vi "Valve_EPICS_Dev4_APX.vi"() -> ()   [LabVIEW 2015]
uses:
  <userlib>/caLab/Private/Get_PV-1D.vi
  <userlib>/caLab/Private/Put_DBL-1D_PV-1D.vi
panel:
  out "Status":bool
  out "Numeric":i32
  out "APX:V7_CLOSE_REQ":bool
  out "APX:V6_CLOSE_REQ":bool
  out "APX:V5_CLOSE_REQ":bool
  out "APX:V4_CLOsE_REQ":bool
  out "AXP:V3_CLOSE_REQ":bool
  out "APX:V2_CLOSE_REQ":bool
  out "APX:V1_CLOSE_REQ":bool
  out "APX:V0_CLOSE_REQ":bool
  out "APX:V7_OPEN_REQ":bool
  out "APX:V6_OPEN_REQ":bool
  out "APX:V5_OPEN_REQ":bool
  out "APX:V4_OPEN_REQ":bool
  out "AXP:V3_OPEN_REQ":bool
  out "APX:V2_OPEN_REQ":bool
  out "APX:V1_OPEN_REQ":bool
  out "APX:V0_OPEN_REQ":bool
  out "APX:V7_OPEN_ENB":bool
  out "APX:V6_OPEN_ENB":bool
  out "APX:V5_OPEN_ENB":bool
  out "APX:V4_OPEN_ENB":bool
  out "APX:V3_OPEN_ENB":bool
  out "APX:V2_OPEN_ENB":bool
  out "APX:V1_OPEN_ENB":bool
  out "APX:V0_OPEN_ENB":bool
  out "Boolean array":bool[](array[boolean])
  out "APX:V7_OPEN_ACT":bool
  out "APX:V6_OPEN_ACT":bool
  out "APX:V5_OPEN_ACT":bool
  out "APX:V4_OPEN_ACT":bool
  out "APX:V3_OPEN_ACT":bool
  out "APX:V2_OPEN_ACT":bool
  out "APX:V1_OPEN_ACT":bool
  out "APX:V0_OPEN_ACT":bool
  out "initialized array":i16[](array[numeric])
  in  "stop":bool
  out "sum":i16
  out "0, 1":i16[](array[numeric])
  out "SCL_data":u32[](array[numeric]) caption="SCL"
  out "SOP_data":u32[](array[numeric]) caption="SOP"
  out "APX:V7_SCL":bool
  out "APX:V6_SCL":bool
  out "APX:V5_SCL":bool
  out "APX:V4_SCL":bool
  out "APX:V3_SCL":bool
  out "APX:V2_SCL":bool
  out "APX:V1_SCL":bool
  out "APX:V0_SCL":bool
  out "APX:V7_SOP":bool
  out "APX:V6_SOP":bool
  out "APX:V5_SOP":bool
  out "APX:V4_SOP":bool
  out "APX:V3_SOP":bool
  out "APX:V2_SOP":bool
  out "APX:V1_SOP":bool
  out "APX:V0_SOP":bool
  # "Valve control DEV4"
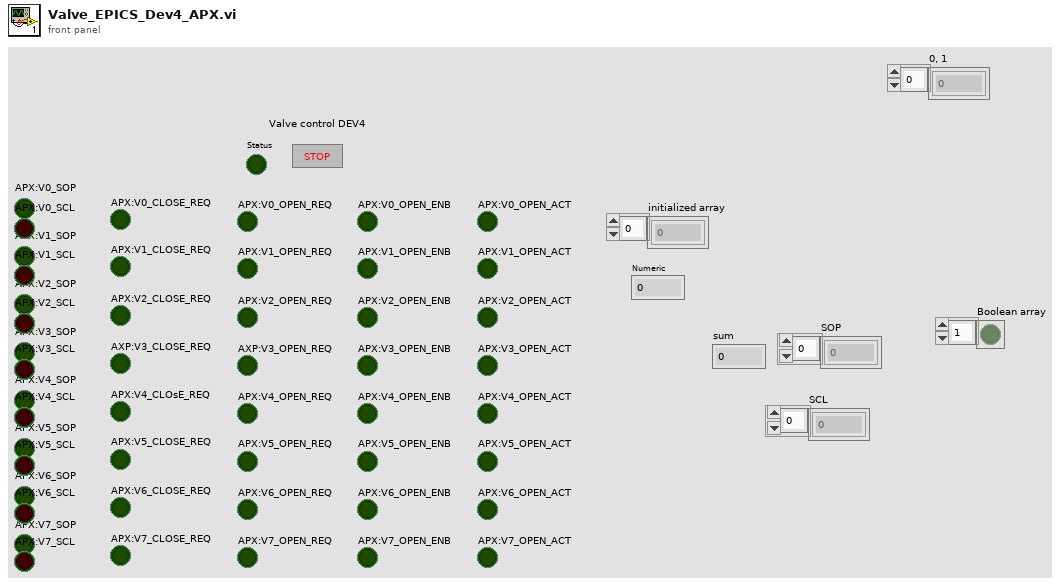
[diagram p1: front panel]
types:
  T1 = typedef "NI_Matrix.lvlib/RealMatrix.ctl" = dbl[][]
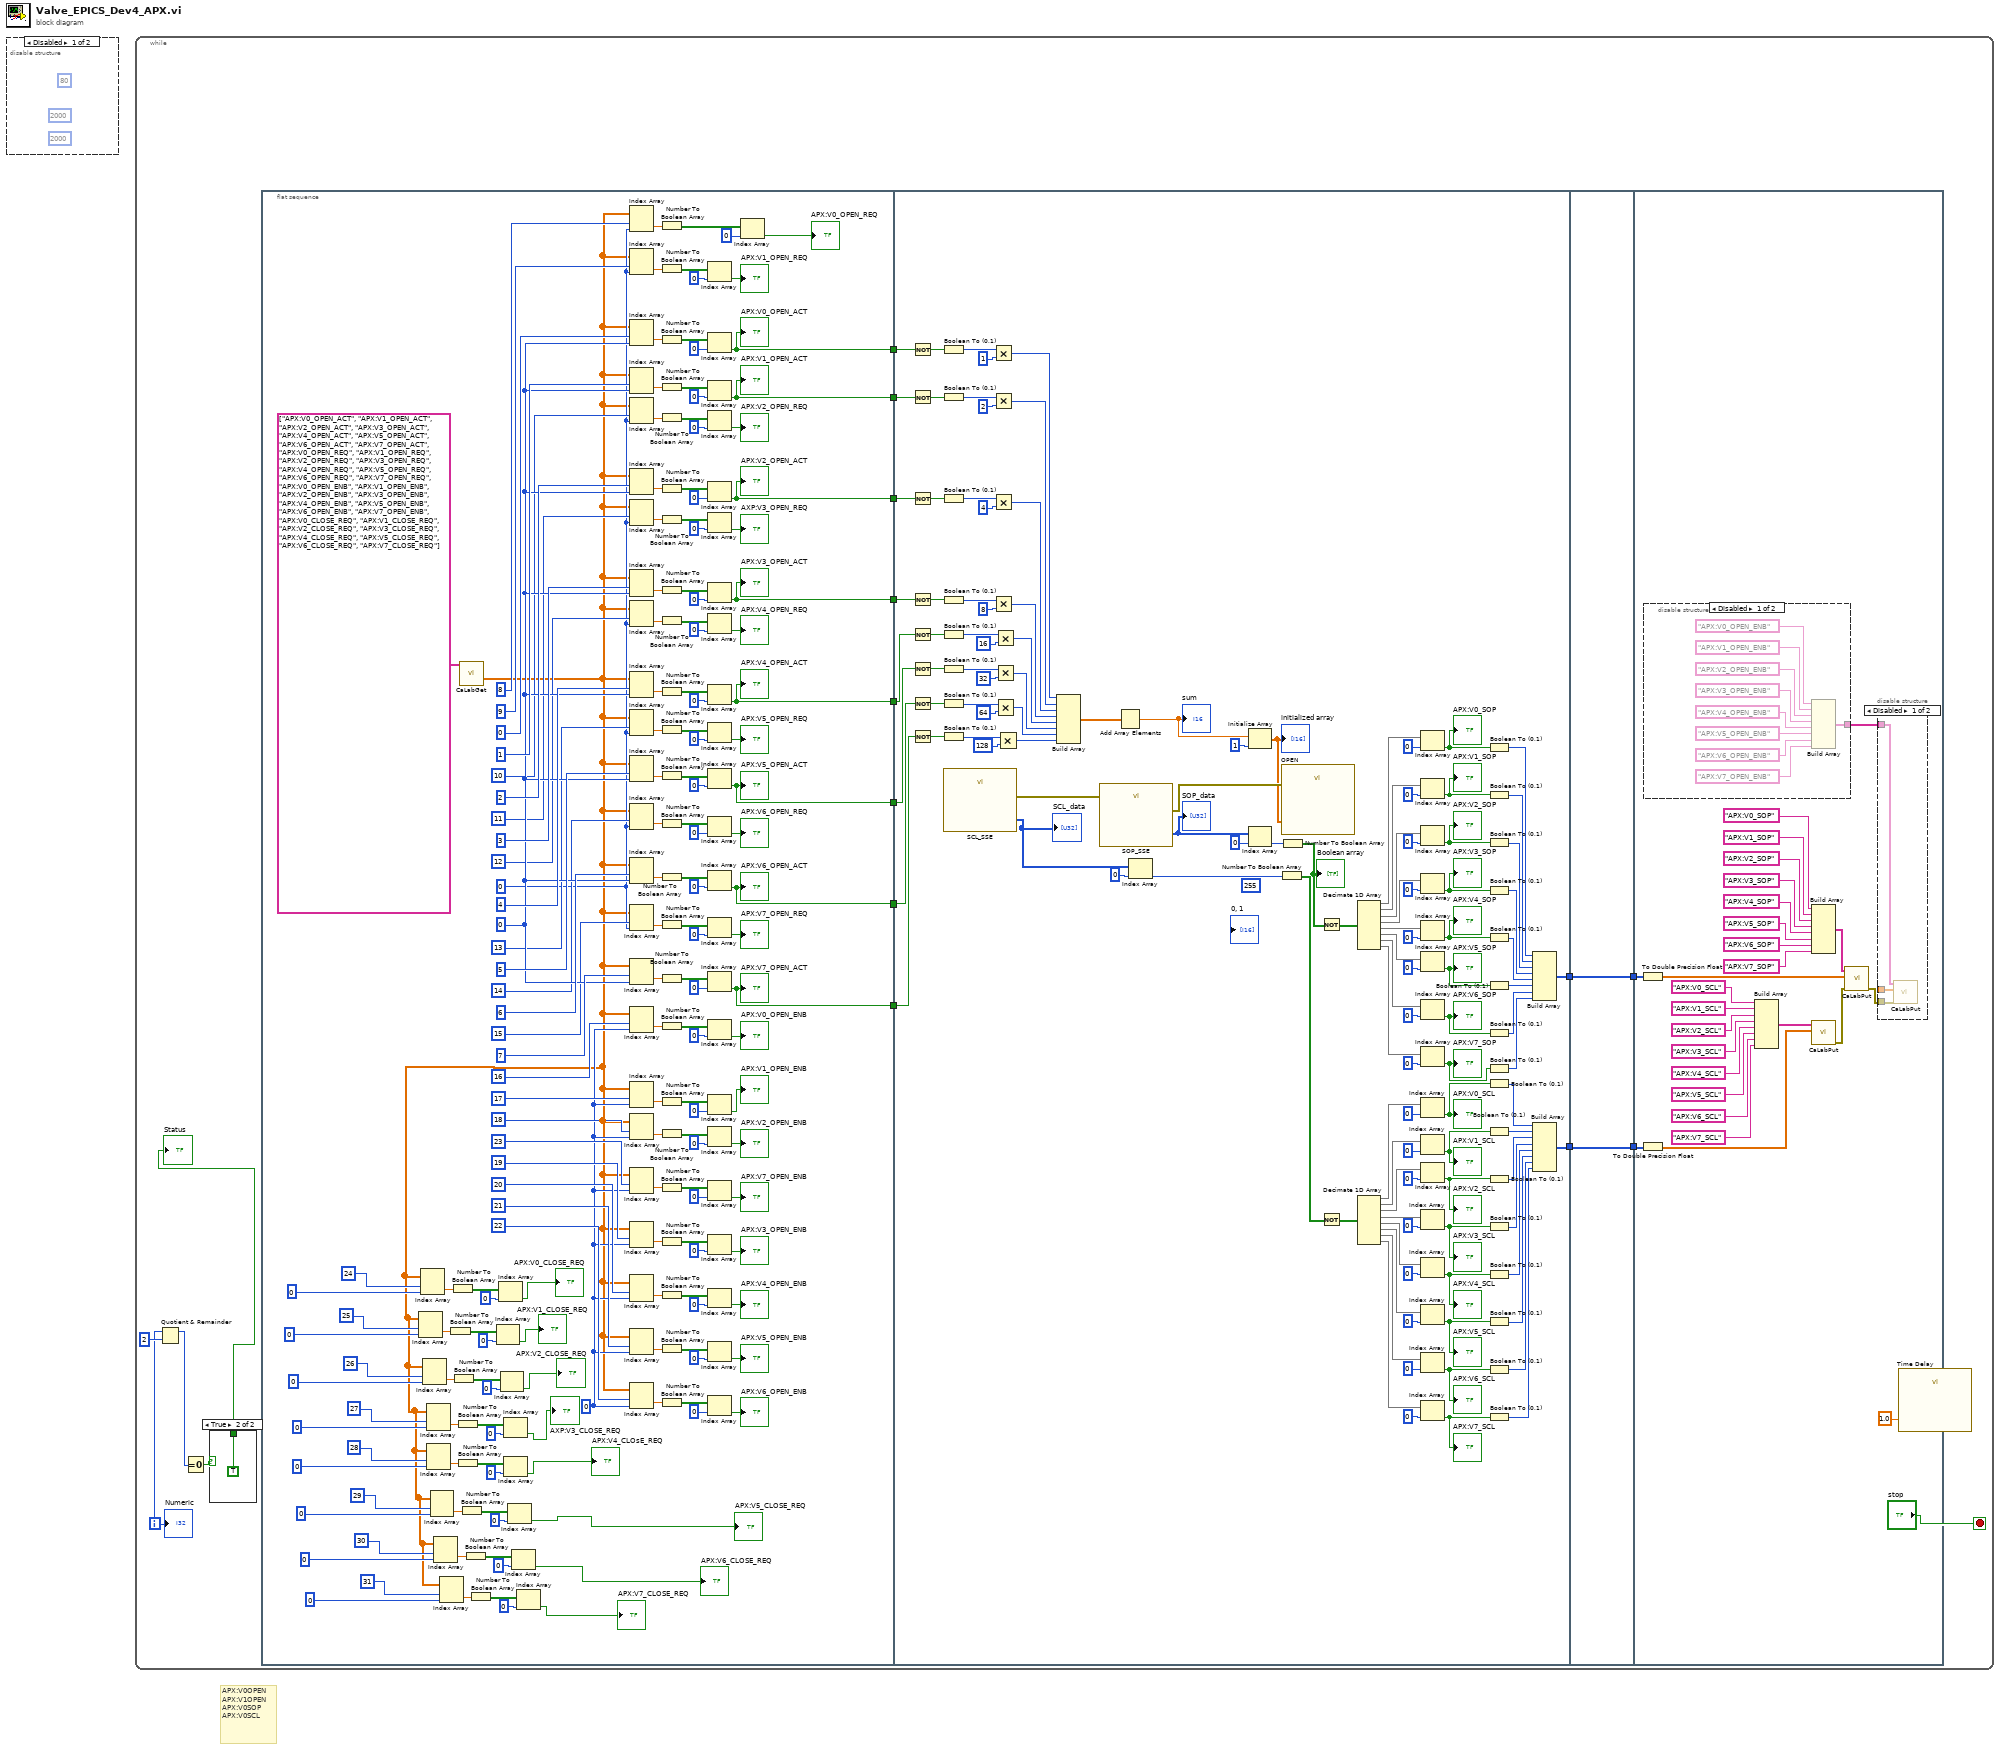
[diagram p0: block diagram]
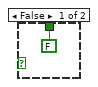
[diagram p3: hidden frame]
diagram:
  # "APX:V0OPEN\nAPX:V1OPEN\nAPX:V0SOP\nAPX:V0SCL"
  n1 = disable-structure shown="Disabled" {
    frame Disabled {
      w1 = 80 ("Priority")
      w2 = 2000 ("Timeout")
      w3 = i64 2000 ("Deadline")
    }
    frame Enabled {
    }
  }
  n2 = while {
    i -> [w5]
    stop <- "stop" stop-if-true
    n3 = Quotient & Remainder(x=w5, y=2) -> (x-y*floor(x/y)=w7:i32)  [unwired: 1 out]
    n4 = Equal To 0?(x=w7) -> (x = 0?=w8:bool)
    n5 = case shown="True" w8 {
      tunnel: [FALSE ("Status") TRUE ("Status")] -> w4
      frame False {
      }
      frame True {
      }
    }
    "Status" <- w4
    n6 = flat-sequence {
      tunnel: [w80] -> w22
      tunnel: [w79] -> w21
      tunnel: [w75] -> w20
      tunnel: [w82] -> w19
      tunnel: [w81] -> w18
      tunnel: [w78] -> w17
      tunnel: [w77] -> w16
      tunnel: [w76] -> w15
      tunnel: w22 -> [w256]
      tunnel: w21 -> [w257]
      tunnel: w20 -> [w258]
      tunnel: w19 -> [w263]
      tunnel: w18 -> [w255]
      tunnel: w17 -> [w259]
      tunnel: w16 -> [w260]
      tunnel: w15 -> [w261]
      tunnel: [w207] -> w14
      tunnel: [w296] -> w11
      tunnel: w14 -> [w321]
      tunnel: [w321] -> w13
      tunnel: w11 -> [w320]
      tunnel: [w320] -> w10
      tunnel: w13 -> [w328]
      tunnel: w10 -> [w326]
      frame #0 {
        w74 = 0 ("index")
        w155 = 0 ("index")
        w188 = 0 ("index")
        n7 = call-poly "CaLabGet.vi"("PV Names"=string[] ["APX:V0_OPEN_ACT", "APX:V1_OPEN_ACT", "APX:V2_OPEN_ACT", "APX:V3_OPEN_ACT", "APX:V4_OPEN_ACT", "APX:V5_OPEN_ACT", "APX:V6_OPEN_ACT", "APX:V7_OPEN_ACT", "APX:V0_OPEN_REQ", "APX:V1_OPEN_REQ", "APX:V2_OPEN_REQ", "APX:V3_OPEN_REQ", "APX:V4_OPEN_REQ", "APX:V5_OPEN_REQ", "APX:V6_OPEN_REQ", "APX:V7_OPEN_REQ", "APX:V0_OPEN_ENB", "APX:V1_OPEN_ENB", "APX:V2_OPEN_ENB", "APX:V3_OPEN_ENB", "APX:V4_OPEN_ENB", "APX:V5_OPEN_ENB", "APX:V6_OPEN_ENB", "APX:V7_OPEN_ENB", "APX:V0_CLOSE_REQ", "APX:V1_CLOSE_REQ", "APX:V2_CLOSE_REQ", "APX:V3_CLOSE_REQ", "APX:V4_CLOSE_REQ", "APX:V5_CLOSE_REQ", "APX:V6_CLOSE_REQ", "APX:V7_CLOSE_REQ"]) -> ("Value Array (number)"=w33:dbl[][])  [unwired: 8 in, 6 out]
        n8 = Index Array(array=w33, index (row)=25 ("index"), index (col)=0 ("index")) -> (element=w66:dbl)
        n9 = Index Array(array=w33, index (row)=24 ("index"), index (col)=0 ("index")) -> (element=w71:dbl)
        n10 = Index Array(array=w33, index (row)=26 ("index"), index (col)=0 ("index")) -> (element=w61:dbl)
        n11 = Index Array(array=w33, index (row)=27 ("index"), index (col)=0 ("index")) -> (element=w56:dbl)
        n12 = Index Array(array=w33, index (row)=28 ("index"), index (col)=0 ("index")) -> (element=w51:dbl)
        n13 = Index Array(array=w33, index (row)=29 ("index"), index (col)=0 ("index")) -> (element=w46:dbl)
        n14 = Index Array(array=w33, index (row)=30 ("index"), index (col)=0 ("index")) -> (element=w41:dbl)
        n15 = Index Array(array=w33, index (row)=31 ("index"), index (col)=0 ("index")) -> (element=w36:dbl)
        n16 = Number To Boolean Array(number=w66) -> (Boolean array=w68:bool[])
        n17 = Number To Boolean Array(number=w71) -> (Boolean array=w73:bool[])
        n18 = Number To Boolean Array(number=w61) -> (Boolean array=w63:bool[])
        n19 = Number To Boolean Array(number=w56) -> (Boolean array=w58:bool[])
        n20 = Number To Boolean Array(number=w51) -> (Boolean array=w53:bool[])
        n21 = Number To Boolean Array(number=w46) -> (Boolean array=w48:bool[])
        n22 = Number To Boolean Array(number=w41) -> (Boolean array=w43:bool[])
        n23 = Number To Boolean Array(number=w36) -> (Boolean array=w38:bool[])
        n24 = Index Array(array=w68, index=0) -> (element=→"APX:V1_CLOSE_REQ":bool)
        n25 = Index Array(array=w73, index=0) -> (element=→"APX:V0_CLOSE_REQ":bool)
        n26 = Index Array(array=w63, index=0) -> (element=→"APX:V2_CLOSE_REQ":bool)
        n27 = Index Array(array=w58, index=0) -> (element=→"AXP:V3_CLOSE_REQ":bool)
        n28 = Index Array(array=w53, index=0) -> (element=→"APX:V4_CLOsE_REQ":bool)
        n29 = Index Array(array=w48, index=0) -> (element=→"APX:V5_CLOSE_REQ":bool)
        n30 = Index Array(array=w43, index=0) -> (element=→"APX:V6_CLOSE_REQ":bool)
        n31 = Index Array(array=w38, index=0) -> (element=→"APX:V7_CLOSE_REQ":bool)
        n32 = Index Array(array=w33, index (row)=8 ("disabled index (row)"), index (col)=w155) -> (element=w135:dbl)
        n33 = Index Array(array=w33, index (row)=9, index (col)=w155) -> (element=w134:dbl)
        n34 = Index Array(array=w33, index (row)=0 ("disabled index (row)"), index (col)=w188) -> (element=w168:dbl)
        n35 = Index Array(array=w33, index (row)=1, index (col)=w188) -> (element=w167:dbl)
        n36 = Index Array(array=w33, index (row)=10, index (col)=w155) -> (element=w138:dbl)
        n37 = Index Array(array=w33, index (row)=2, index (col)=w188) -> (element=w171:dbl)
        n38 = Index Array(array=w33, index (row)=11 ("index"), index (col)=w155) -> (element=w137:dbl)
        n39 = Index Array(array=w33, index (row)=3 ("index"), index (col)=w188) -> (element=w170:dbl)
        n40 = Index Array(array=w33, index (row)=12, index (col)=w155) -> (element=w136:dbl)
        n41 = Index Array(array=w33, index (row)=4, index (col)=w188) -> (element=w169:dbl)
        n42 = Index Array(array=w33, index (row)=13, index (col)=w155) -> (element=w133:dbl)
        n43 = Index Array(array=w33, index (row)=5, index (col)=w188) -> (element=w166:dbl)
        n44 = Index Array(array=w33, index (row)=14, index (col)=w155) -> (element=w132:dbl)
        n45 = Index Array(array=w33, index (row)=6, index (col)=w188) -> (element=w165:dbl)
        n46 = Index Array(array=w33, index (row)=15, index (col)=w155) -> (element=w131:dbl)
        n47 = Index Array(array=w33, index (row)=7, index (col)=w188) -> (element=w164:dbl)
        n48 = Index Array(array=w33, index (row)=16 ("disabled index (row)"), index (col)=w74) -> (element=w103:dbl)
        n49 = Index Array(array=w33, index (row)=17, index (col)=w74) -> (element=w102:dbl)
        n50 = Index Array(array=w33, index (row)=18, index (col)=w74) -> (element=w106:dbl)
        n51 = Index Array(array=w33, index (row)=23, index (col)=w74) -> (element=w99:dbl)
        n52 = Index Array(array=w33, index (row)=19 ("index"), index (col)=w74) -> (element=w105:dbl)
        n53 = Index Array(array=w33, index (row)=20, index (col)=w74) -> (element=w104:dbl)
        n54 = Index Array(array=w33, index (row)=21, index (col)=w74) -> (element=w101:dbl)
        n55 = Index Array(array=w33, index (row)=22, index (col)=w74) -> (element=w100:dbl)
        n56 = Number To Boolean Array(number=w135) -> (Boolean array=w148:bool[])
        n57 = Number To Boolean Array(number=w134) -> (Boolean array=w146:bool[])
        n58 = Number To Boolean Array(number=w168) -> (Boolean array=w181:bool[])
        n59 = Number To Boolean Array(number=w167) -> (Boolean array=w179:bool[])
        n60 = Number To Boolean Array(number=w138) -> (Boolean array=w154:bool[])
        n61 = Number To Boolean Array(number=w171) -> (Boolean array=w187:bool[])
        n62 = Number To Boolean Array(number=w137) -> (Boolean array=w152:bool[])
        n63 = Number To Boolean Array(number=w170) -> (Boolean array=w185:bool[])
        n64 = Number To Boolean Array(number=w136) -> (Boolean array=w150:bool[])
        n65 = Number To Boolean Array(number=w169) -> (Boolean array=w183:bool[])
        n66 = Number To Boolean Array(number=w133) -> (Boolean array=w144:bool[])
        n67 = Number To Boolean Array(number=w166) -> (Boolean array=w177:bool[])
        n68 = Number To Boolean Array(number=w132) -> (Boolean array=w142:bool[])
        n69 = Number To Boolean Array(number=w165) -> (Boolean array=w175:bool[])
        n70 = Number To Boolean Array(number=w131) -> (Boolean array=w140:bool[])
        n71 = Number To Boolean Array(number=w164) -> (Boolean array=w173:bool[])
        n72 = Number To Boolean Array(number=w103) -> (Boolean array=w116:bool[])
        n73 = Number To Boolean Array(number=w102) -> (Boolean array=w114:bool[])
        n74 = Number To Boolean Array(number=w106) -> (Boolean array=w122:bool[])
        n75 = Number To Boolean Array(number=w99) -> (Boolean array=w108:bool[])
        n76 = Number To Boolean Array(number=w105) -> (Boolean array=w120:bool[])
        n77 = Number To Boolean Array(number=w104) -> (Boolean array=w118:bool[])
        n78 = Number To Boolean Array(number=w101) -> (Boolean array=w112:bool[])
        n79 = Number To Boolean Array(number=w100) -> (Boolean array=w110:bool[])
        n80 = Index Array(array=w146, index=0) -> (element=→"APX:V1_OPEN_REQ":bool)
        n81 = Index Array(array=w181, index=0) -> (element=w82:bool)
        "APX:V0_OPEN_ACT" <- w82
        n82 = Index Array(array=w179, index=0) -> (element=w81:bool)
        "APX:V1_OPEN_ACT" <- w81
        n83 = Index Array(array=w154, index=0) -> (element=→"APX:V2_OPEN_REQ":bool)
        n84 = Index Array(array=w187, index=0) -> (element=w80:bool)
        "APX:V2_OPEN_ACT" <- w80
        n85 = Index Array(array=w152, index=0) -> (element=→"AXP:V3_OPEN_REQ":bool)
        n86 = Index Array(array=w185, index=0) -> (element=w79:bool)
        "APX:V3_OPEN_ACT" <- w79
        n87 = Index Array(array=w150, index=0) -> (element=→"APX:V4_OPEN_REQ":bool)
        n88 = Index Array(array=w183, index=0) -> (element=w75:bool)
        "APX:V4_OPEN_ACT" <- w75
        n89 = Index Array(array=w144, index=0) -> (element=→"APX:V5_OPEN_REQ":bool)
        n90 = Index Array(array=w177, index=0) -> (element=w78:bool)
        "APX:V5_OPEN_ACT" <- w78
        n91 = Index Array(array=w142, index=0) -> (element=→"APX:V6_OPEN_REQ":bool)
        n92 = Index Array(array=w175, index=0) -> (element=w77:bool)
        "APX:V6_OPEN_ACT" <- w77
        n93 = Index Array(array=w140, index=0) -> (element=→"APX:V7_OPEN_REQ":bool)
        n94 = Index Array(array=w173, index=0) -> (element=w76:bool)
        "APX:V7_OPEN_ACT" <- w76
        n95 = Index Array(array=w116, index=0) -> (element=→"APX:V0_OPEN_ENB":bool)
        n96 = Index Array(array=w114, index=0) -> (element=→"APX:V1_OPEN_ENB":bool)
        n97 = Index Array(array=w122, index=0) -> (element=→"APX:V2_OPEN_ENB":bool)
        n98 = Index Array(array=w108, index=0) -> (element=→"APX:V7_OPEN_ENB":bool)
        n99 = Index Array(array=w120, index=0) -> (element=→"APX:V3_OPEN_ENB":bool)
        n100 = Index Array(array=w118, index=0) -> (element=→"APX:V4_OPEN_ENB":bool)
        n101 = Index Array(array=w112, index=0) -> (element=→"APX:V5_OPEN_ENB":bool)
        n102 = Index Array(array=w110, index=0) -> (element=→"APX:V6_OPEN_ENB":bool)
        n103 = Index Array "Index Array"(array=w148, index=0) -> (element=→"APX:V0_OPEN_REQ":bool)
      }
      frame #1 {
        (unwired) u32 255 ("y")
        n104 = Not(x=w263) -> (.not. x?=w262:bool)
        n105 = Not(x=w255) -> (.not. x?=w287:bool)
        n106 = Not(x=w256) -> (.not. x?=w286:bool)
        n107 = Not(x=w257) -> (.not. x?=w285:bool)
        n108 = Not(x=w258) -> (.not. x?=w284:bool)
        n109 = Not(x=w259) -> (.not. x?=w283:bool)
        n110 = Not(x=w260) -> (.not. x?=w282:bool)
        n111 = Not(x=w261) -> (.not. x?=w281:bool)
        n112 = Boolean To (0,1)(Boolean=w262) -> (0, 1=w295:i16)
        n113 = Boolean To (0,1)(Boolean=w287) -> (0, 1=w294:i16)
        n114 = Boolean To (0,1)(Boolean=w286) -> (0, 1=w293:i16)
        n115 = Boolean To (0,1)(Boolean=w285) -> (0, 1=w292:i16)
        n116 = Boolean To (0,1)(Boolean=w284) -> (0, 1=w291:i16)
        n117 = Boolean To (0,1)(Boolean=w283) -> (0, 1=w290:i16)
        n118 = Boolean To (0,1)(Boolean=w282) -> (0, 1=w289:i16)
        n119 = Boolean To (0,1)(Boolean=w281) -> (0, 1=w288:i16)
        n120 = call "SCL_SSE"() -> ("data"=w235:u32[], "error out"=w310:errorcluster)  [unwired: 17 in, 1 out]
        "SCL_data" <- w235
        n121 = Multiply(x=w295, y=i16 1) -> (x*y=w272:i16)
        n122 = Multiply(x=w294, y=i16 2) -> (x*y=w271:i16)
        n123 = Multiply(x=w293, y=i16 4) -> (x*y=w270:i16)
        n124 = Multiply(x=w292, y=i16 8) -> (x*y=w269:i16)
        n125 = Multiply(x=w291, y=i16 16) -> (x*y=w268:i16)
        n126 = Multiply(x=w290, y=i16 32) -> (x*y=w267:i16)
        n127 = Multiply(x=w289, y=i16 64) -> (x*y=w266:i16)
        n128 = Multiply(x=w288, y=i16 128) -> (x*y=w265:i16)
        n129 = Build Array(w272, w271, w270, w269, w268, w267, w266, w265) -> (w264:T1)
        n130 = call "SOP_SSE"("error in"=w310) -> ("data"=w234:u32[], "error out"=w309:errorcluster)  [unwired: 16 in, 1 out]
        "SOP_data" <- w234
        n131 = Add Array Elements(numeric array=w264) -> (sum=w307:dbl)
        "sum" <- w307
        n132 = Index Array(array=w235, index=0) -> (element=w253:u32)
        n133 = Initialize Array(w307, 1 ("dimension size")) -> (w306:dbl[])
        "initialized array" <- w306
        n134 = Index Array(array=w234, index=0) -> (element=w254:u32)
        n135 = Number To Boolean Array(number=w253) -> (Boolean array=w244:bool[])
        n136 = call "OPEN"("data"=w306, "error in"=w309) -> ()  [unwired: 16 in, 2 out]
        n137 = Number To Boolean Array(number=w254) -> (Boolean array=w233:bool[])
        "Boolean array" <- w233
        n138 = Not(x=w233) -> (.not. x?=w232:bool[])
        n139 = Not(x=w244) -> (.not. x?=w231:bool[])
        n140 = Decimate 1D Array(w232) -> (w252:bool[], w251:bool[], w250:bool[], w249:bool[], w248:bool[], w247:bool[], w246:bool[], w245:bool[])
        n141 = Decimate 1D Array(w231) -> (w243:bool[], w242:bool[], w241:bool[], w240:bool[], w239:bool[], w238:bool[], w237:bool[], w236:bool[])
        n142 = Index Array(array=w252, index=0) -> (element=w215:bool)
        "APX:V0_SOP" <- w215
        n143 = Index Array(array=w251, index=0) -> (element=w230:bool)
        "APX:V1_SOP" <- w230
        n144 = Index Array(array=w250, index=0) -> (element=w222:bool)
        "APX:V2_SOP" <- w222
        n145 = Index Array(array=w249, index=0) -> (element=w221:bool)
        "APX:V3_SOP" <- w221
        n146 = Index Array(array=w248, index=0) -> (element=w220:bool)
        "APX:V4_SOP" <- w220
        n147 = Index Array(array=w247, index=0) -> (element=w219:bool)
        "APX:V5_SOP" <- w219
        n148 = Index Array(array=w246, index=0) -> (element=w218:bool)
        "APX:V6_SOP" <- w218
        n149 = Index Array(array=w245, index=0) -> (element=w217:bool)
        "APX:V7_SOP" <- w217
        n150 = Index Array(array=w243, index=0) -> (element=w205:bool)
        "APX:V0_SCL" <- w205
        n151 = Index Array(array=w242, index=0) -> (element=w204:bool)
        "APX:V1_SCL" <- w204
        n152 = Index Array(array=w241, index=0) -> (element=w203:bool)
        "APX:V2_SCL" <- w203
        n153 = Index Array(array=w240, index=0) -> (element=w202:bool)
        "APX:V3_SCL" <- w202
        n154 = Index Array(array=w239, index=0) -> (element=w201:bool)
        "APX:V4_SCL" <- w201
        n155 = Index Array(array=w238, index=0) -> (element=w200:bool)
        "APX:V5_SCL" <- w200
        n156 = Index Array(array=w237, index=0) -> (element=w199:bool)
        "APX:V6_SCL" <- w199
        n157 = Index Array(array=w236, index=0) -> (element=w198:bool)
        "APX:V7_SCL" <- w198
        n158 = Boolean To (0,1)(Boolean=w215) -> (0, 1=w216:i16)
        n159 = Boolean To (0,1)(Boolean=w230) -> (0, 1=w229:i16)
        n160 = Boolean To (0,1)(Boolean=w222) -> (0, 1=w228:i16)
        n161 = Boolean To (0,1)(Boolean=w221) -> (0, 1=w227:i16)
        n162 = Boolean To (0,1)(Boolean=w220) -> (0, 1=w226:i16)
        n163 = Boolean To (0,1)(Boolean=w219) -> (0, 1=w225:i16)
        n164 = Boolean To (0,1)(Boolean=w218) -> (0, 1=w224:i16)
        n165 = Boolean To (0,1)(Boolean=w217) -> (0, 1=w223:i16)
        n166 = Boolean To (0,1)(Boolean=w205) -> (0, 1=w208:i16)
        n167 = Boolean To (0,1)(Boolean=w204) -> (0, 1=w214:i16)
        n168 = Boolean To (0,1)(Boolean=w203) -> (0, 1=w213:i16)
        n169 = Boolean To (0,1)(Boolean=w202) -> (0, 1=w212:i16)
        n170 = Boolean To (0,1)(Boolean=w201) -> (0, 1=w211:i16)
        n171 = Boolean To (0,1)(Boolean=w200) -> (0, 1=w210:i16)
        n172 = Boolean To (0,1)(Boolean=w199) -> (0, 1=w209:i16)
        n173 = Boolean To (0,1)(Boolean=w198) -> (0, 1=w206:i16)
        n174 = Build Array(w216, w229, w228, w227, w226, w225, w224, w223) -> (w296:i16[])
        n175 = Build Array(w208, w214, w213, w212, w211, w210, w209, w206) -> (w207:i16[])
      }
      frame #2 {
      }
      frame #3 {
        n176 = To Double Precision Float(number=w326) -> (double precision float=w329:dbl[])
        n177 = To Double Precision Float(number=w328) -> (double precision float=w327:dbl[])
        n178 = disable-structure shown="Disabled" {
          disable-tunnel: [w350 _] -> w324
          frame Disabled {
            n179 = Build Array("APX:V0_OPEN_ENB", "APX:V1_OPEN_ENB", "APX:V2_OPEN_ENB", "APX:V3_OPEN_ENB", "APX:V4_OPEN_ENB", "APX:V5_OPEN_ENB", "APX:V6_OPEN_ENB", "APX:V7_OPEN_ENB") -> (w350:string[])
          }
          frame Enabled {
          }
        }
        n180 = Build Array("APX:V0_SCL", "APX:V1_SCL", "APX:V2_SCL", "APX:V3_SCL", "APX:V4_SCL", "APX:V5_SCL", "APX:V6_SCL", "APX:V7_SCL") -> (w330:string[])
        n181 = Build Array("APX:V0_SOP", "APX:V1_SOP", "APX:V2_SOP", "APX:V3_SOP", "APX:V4_SOP", "APX:V5_SOP", "APX:V6_SOP", "APX:V7_SOP") -> (w325:string[])
        n182 = call-poly <userlib>:"CaLabPut.vi"("Values"=w327, "PV Names"=w330) -> ("Error out"=w322:errorcluster)  [unwired: 6 in, 3 out]
        n183 = call-poly <userlib>:"CaLabPut.vi"("Error in (no error)"=w322, "Values"=w329, "PV Names"=w325) -> ("Error out"=w323:errorcluster)  [unwired: 5 in, 3 out]
        n184 = disable-structure shown="Disabled" {
          disable-tunnel: _ -> [w349 _]
          disable-tunnel: w324 -> [w348 _]
          disable-tunnel: w323 -> [w347 _]
          frame Disabled {
            n185 = call-poly <userlib>:"CaLabPut.vi"("Error in (no error)"=w347, "Values"=w349, "PV Names"=w348) -> ()  [unwired: 5 in, 4 out]
          }
          frame Enabled {
          }
        }
      }
    }
    n186 = call "Time Delay"("Delay Time (s)"=1.0) -> ()  [unwired: 10 in, 1 out]
    "Numeric" <- w5
  }
